vi "BytesPerReadout (SubVI).vi"(9 "DataAcquisitionBuffer in":T1) -> (0 "Bytes per ROI":i32[](array[numeric]), 1 "Metadata Bytes":i32, 3 "Bytes/Readout >":i32)   [LabVIEW 2019, in "PICam.lvlib"]
uses:
  PICam.lvlib
  types/utility/DataAcquisitionResult.ctl
  types/PicamRoi.ctl
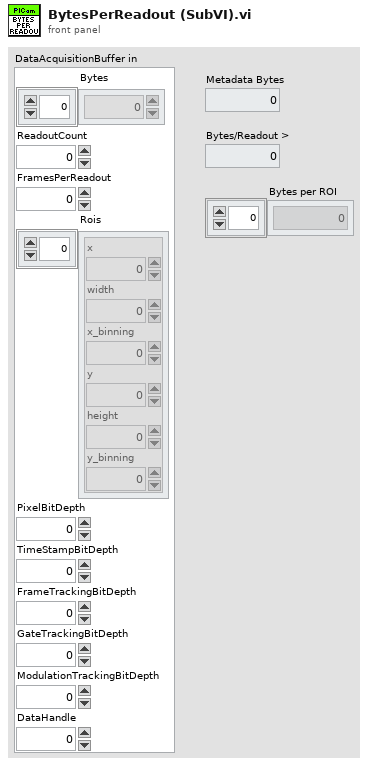
[diagram p1: front panel]
types:
  T1 = typedef "PICam.lvlib/DataAcquisitionResult.ctl" = cluster{"Bytes":u8[], "ReadoutCount":i64, "FramesPerReadout":i32, "Rois":T2[], "PixelBitDepth":i32, "TimeStampBitDepth":i32, "FrameTrackingBitDepth":i32, "GateTrackingBitDepth":i32, "ModulationTrackingBitDepth":i32, "DataHandle":u64}
  T2 = typedef "PicamRoi.ctl" = cluster{"x":i32, "width":i32, "x_binning":i32, "y":i32, "height":i32, "y_binning":i32}
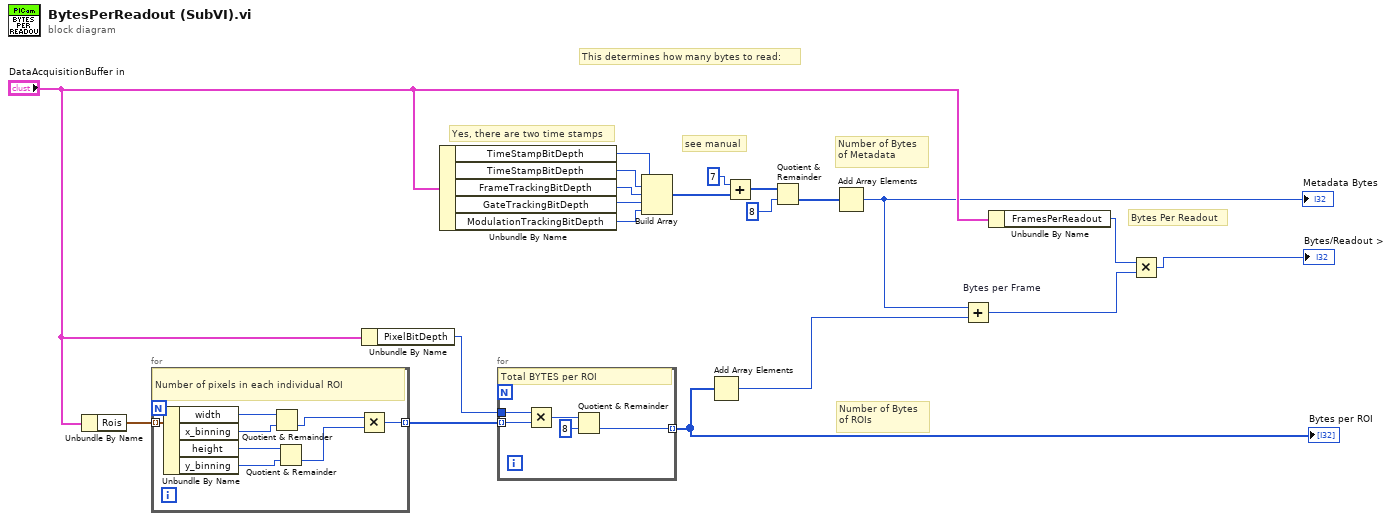
[diagram p0: block diagram]
diagram:
  # "Bytes Per Readout"
  # "Number of Bytes\nof ROIs"
  # "This determines how many bytes to read:"
  # "see manual"
  # "Yes, there are two time stamps"
  # "Number of Bytes\nof Metadata"
  n1 = Unbundle By Name("DataAcquisitionBuffer in") -> ("Rois"=w3:T2[])
  n2 = for {
    tunnel: [w28] -> w1 mode=indexing
    tunnel: w3 -> [w27] mode=indexing
    # "Number of pixels in each individual ROI"
    n3 = Unbundle By Name(w27) -> ("width"=w26:i32, "x_binning"=w25:i32, "height"=w24:i32, "y_binning"=w22:i32)
    n4 = Quotient & Remainder(x=w26, y=w25) -> (floor(x/y)=w23:i32)  [unwired: 1 out]
    n5 = Quotient & Remainder(x=w24, y=w22) -> (floor(x/y)=w21:i32)  [unwired: 1 out]
    n6 = Multiply(x=w23, y=w21) -> (x*y=w28:i32)
  }
  n7 = Unbundle By Name("DataAcquisitionBuffer in") -> ("PixelBitDepth"=w4:i32)
  n8 = Unbundle By Name("DataAcquisitionBuffer in") -> ("TimeStampBitDepth"=w10:i32, "TimeStampBitDepth"=w5:i32, "FrameTrackingBitDepth"=w8:i32, "GateTrackingBitDepth"=w7:i32, "ModulationTrackingBitDepth"=w6:i32)
  n9 = for {
    tunnel: w1 -> [w33] mode=indexing
    tunnel: [w30] -> w2 mode=indexing
    tunnel: w4 -> [w29]
    # "Total BYTES per ROI"
    n10 = Multiply(x=w29, y=w33) -> (x*y=w32:i32)
    n11 = Quotient & Remainder(x=w32, y=8) -> (floor(x/y)=w30:i32)  [unwired: 1 out]
  }
  "Bytes per ROI" <- w2
  n12 = Build Array(w10, w5, w8, w7, w6) -> (w9:i32[])
  n13 = Add Array Elements(numeric array=w2) -> (sum=w16:i32)
  n14 = Add(x=7, y=w9) -> (x+y=w12:i32[])
  n15 = Quotient & Remainder(x=w12, y=8) -> (floor(x/y)=w14:i32[])  [unwired: 1 out]
  n16 = Add Array Elements(numeric array=w14) -> (sum=w15:i32)
  "Metadata Bytes" <- w15
  n17 = Add "Bytes per Frame"(x=w15, y=w16) -> (x+y=w18:i32)
  n18 = Unbundle By Name("DataAcquisitionBuffer in") -> ("FramesPerReadout"=w17:i32)
  n19 = Multiply(x=w17, y=w18) -> (x*y=→"Bytes/Readout >":i32)
